vi "NXT_MIDBRAIN Read NXTBEE.vi"(3 "error in (no error)":errorcluster, 4 "#bytes":u8) -> (0 "error out":errorcluster, 1 "Valid String?":bool, 2 "Data Out":u8[](array[numeric]))   [LabVIEW 2012]
doc: "Description:\nThis VI reads the specified number of bytes from the NXTBee sensor. \n\nInputs:\n-Number of bytes to be read during each read operation.\n-Error wire in\n\nOutputs:\n-Byte array of character data\n-Error wire out"
uses:
  <vilib>/NXT/NXT Controls/NXTSyscallRefnum.ctl
  <resource>/objmgr/NXTInputOutput.rc
panel:
  out "Numeric":i32
  out "Refnum Out":T1
  in  "Sys Call Refnum":T1
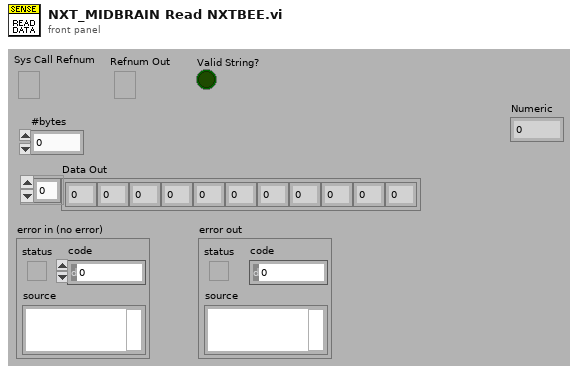
[diagram p1: front panel]
types:
  T1 = typedef "NXTSyscallRefnum.ctl" = refnum<k21>
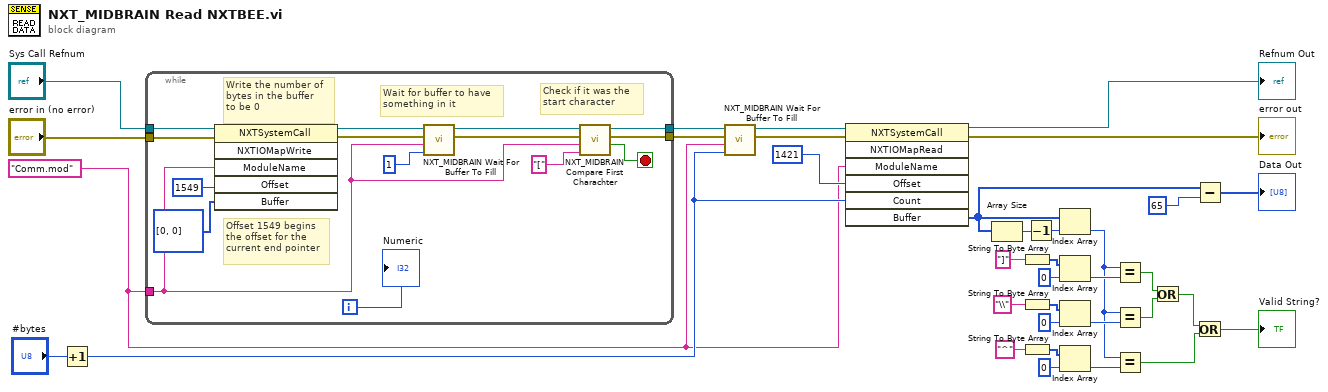
[diagram p0: block diagram]
diagram:
  w4 = "Comm.mod" ("ModuleName")
  n1 = Increment(x="#bytes") -> (x+1=w7:u8)
  n2 = while {
    tunnel: w4 -> [w36]
    tunnel: [w45] -> w11
    tunnel: [w44] -> w10
    tunnel: "error in (no error)" -> [w38]
    tunnel: "Sys Call Refnum" -> [w37]
    i -> [w43]
    stop <- w46 stop-if-true
    # "Write the number of\nbytes in the buffer\nto be 0"
    # "Offset 1549 begins\nthe offset for the\ncurrent end pointer"
    # "Check if it was the \nstart character"
    # "Wait for buffer to have\nsomething in it"
    n3 = invoke class="NXTSystemCall" method="NXTIOMapWrite"(reference=w37, error in=w38, "ModuleName"=w36, "Offset"=u16 1549, "Buffer"=u8[] [0, 0]) -> (reference out=w40:T1, error out=w39:errorcluster)  [unwired: 1 in, 4 out]
    n4 = call "NXT_MIDBRAIN Wait For Buffer To Fill.vi"("Buffer Length"=u8 1 ("x"), "ModuleName"=w36, "error in (no error)"=w39, "Refnum in"=w40) -> ("error out"=w48:errorcluster, "Refnum out"=w49:T1)  [unwired: 2 in]
    n5 = call "NXT_MIDBRAIN Compare First Charachter.vi"("string"="[", "ModuleName"=w36, "error in (no error)"=w48, "Refnum in"=w49) -> ("Boolean"=w46:bool, "error out"=w44:errorcluster, "Refnum Out"=w45:T1)  [unwired: 1 in]
    "Numeric" <- w43
  }
  n6 = call "NXT_MIDBRAIN Wait For Buffer To Fill.vi"("Buffer Length"=w7, "ModuleName"=w4, "error in (no error)"=w10, "Refnum in"=w11) -> ("error out"=w8:errorcluster, "Refnum out"=w9:T1)  [unwired: 2 in]
  n7 = invoke class="NXTSystemCall" method="NXTIOMapRead"(reference=w9, error in=w8, "ModuleName"=w4, "Offset"=u16 1421, "Count"=w7) -> (reference out=→"Refnum Out":T1, error out=→"error out":errorcluster, "Buffer"=w3:u8[])  [unwired: 2 in, 4 out]
  n8 = Array Size(array=w3) -> (size(s)=w30:i32)
  n9 = String To Byte Array(string="]") -> (unsigned byte array=w28:u8[])
  n10 = String To Byte Array(string="\\") -> (unsigned byte array=w25:u8[])
  n11 = String To Byte Array(string="^") -> (unsigned byte array=w22:u8[])
  n12 = Decrement(x=w30) -> (x-1=w31:i32)
  n13 = Index Array(array=w3, index=w31) -> (element=w17:u8)
  n14 = Index Array(array=w28, index=0) -> (element=w20:u8)
  n15 = Index Array(array=w25, index=0) -> (element=w18:u8)
  n16 = Index Array(array=w22, index=0) -> (element=w19:u8)
  n17 = Equal?(x=w17, y=w20) -> (x = y?=w15:bool)
  n18 = Equal?(x=w17, y=w18) -> (x = y?=w16:bool)
  n19 = Equal?(x=w17, y=w19) -> (x = y?=w13:bool)
  n20 = Or(x=w15, y=w16) -> (x .or. y?=w14:bool)
  n21 = Subtract(x=w3, y=u8 65) -> (x-y=→"Data Out":u8[])
  n22 = Or(x=w14, y=w13) -> (x .or. y?=→"Valid String?":bool)
